vi "GEOM_findAmplifierbyCoordMult.vi"(7 "mode":enum16{"=", "<", ">", "<=", ">="}(ring), 9 "amplifiers":T1[](array[typedef]) {"fliped" items=["none", "horizontal", "vertical"]; "type" items=["LL", "LR", "UL", "UR"]}, 10 "ycoord":i32, 11 "xcoord":i32) -> (1 "amplifiers":T1[](array[typedef]) {"fliped" items=["none", "horizontal", "vertical"]; "type" items=["LL", "LR", "UL", "UR"]}, 2 "indexes":i32[](array[numeric]))   [LabVIEW 2016]
uses:
  GEOM_Amplifier.ctl
  GEOM_AmpType.ctl
  GEOM_ROI.ctl
  GEOM_Coords.ctl
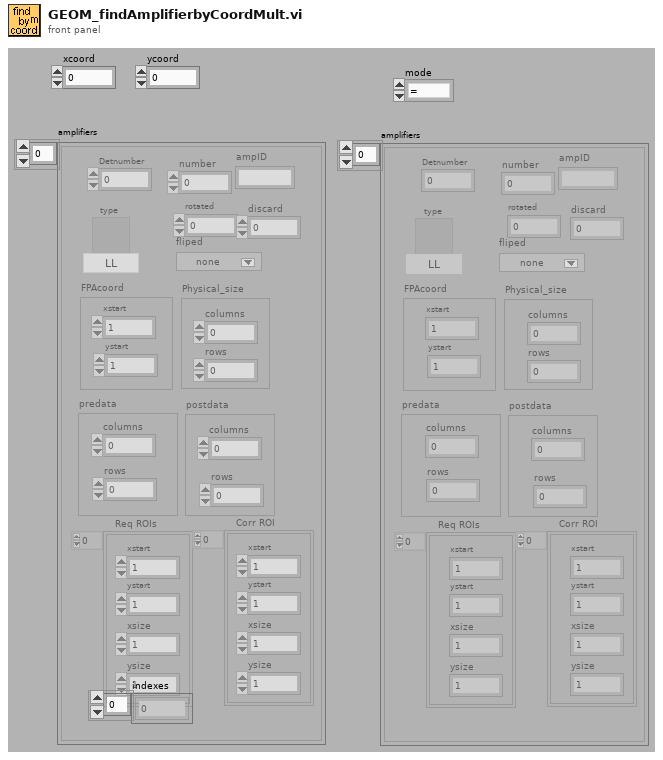
[diagram p1: front panel]
types:
  T1 = typedef "GEOM_Amplifier.ctl" = cluster{"number":i32, "type":T2, "rotated":i16, "fliped":u16, "FPAcoord":cluster{"xstart":i32, "ystart":i32}, "Physical_size":cluster{"columns":i32, "rows":i32}, "predata":cluster{"columns":i32, "rows":i32}, "postdata":cluster{"columns":i32, "rows":i32}, "Req ROIs":T3, "Corr ROI":T3, "Detnumber":i32, "ampID":string, "discard":i32}
  T2 = typedef "GEOM_AmpType.ctl" = u16
  T3 = typedef "GEOM_ROI.ctl" = T4[]
  T4 = typedef "GEOM_Coords.ctl" = cluster{"xstart":u32, "ystart":u32, "xsize":u32, "ysize":u32}
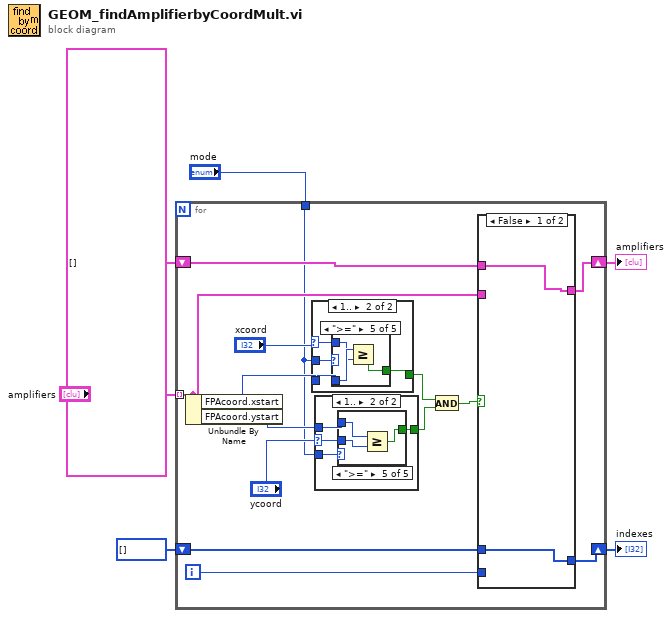
[diagram p0: block diagram]
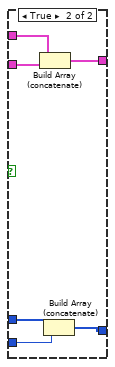
[diagram p2: hidden frame]
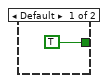
[diagram p3: hidden frame]
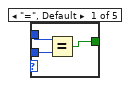
[diagram p4: hidden frame]
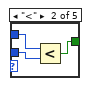
[diagram p5: hidden frame]
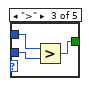
[diagram p6: hidden frame]
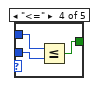
[diagram p7: hidden frame]
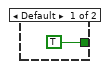
[diagram p8: hidden frame]
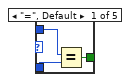
[diagram p9: hidden frame]
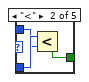
[diagram p10: hidden frame]
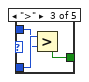
[diagram p11: hidden frame]
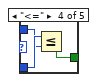
[diagram p12: hidden frame]
diagram:
  n1 = for {
    tunnel: "amplifiers" -> [w13] mode=indexing
    shift-right: [w12] -> w5
    shift-left: T1[] [] -> [w11]
    shift-right: [w9] -> w4
    shift-left: i32[] [] -> [w8]
    tunnel: "mode" -> [w7]
    i -> [w10]
    n2 = Unbundle By Name(w13) -> ("FPAcoord.xstart"=w20:i32, "FPAcoord.ystart"=w19:i32)
    n3 = case shown="1.." "xcoord" {
      selector: "xcoord" -> [_ w51]
      tunnel: w20 -> [_ w53]
      tunnel: [TRUE w52] -> w18
      tunnel: w7 -> [_ w50]
      frame Default {
      }
      frame 1.. {
        n4 = case shown="\">=\"" w50 {
          tunnel: w53 -> [w56 w58 w61 w64 w67]
          tunnel: [w55 w59 w62 w65 w68] -> w52
          tunnel: w51 -> [w54 w57 w60 w63 w66]
          frame "=", Default {
            n5 = Equal?(x=w54, y=w56) -> (x = y?=w55:bool)
          }
          frame "<" {
            n6 = Less?(x=w58, y=w57) -> (x < y?=w59:bool)
          }
          frame ">" {
            n7 = Greater?(x=w61, y=w60) -> (0:w62:bool)
          }
          frame "<=" {
            n8 = Less Or Equal?(x=w64, y=w63) -> (x <= y?=w65:bool)
          }
          frame ">=" {
            n9 = Greater Or Equal?(x=w67, y=w66) -> (x >= y?=w68:bool)
          }
        }
      }
    }
    n10 = case shown="1.." "ycoord" {
      selector: "ycoord" -> [_ w31]
      tunnel: w19 -> [_ w33]
      tunnel: [TRUE w32] -> w17
      tunnel: w7 -> [_ w30]
      frame Default {
      }
      frame 1.. {
        n11 = case shown="\">=\"" w30 {
          tunnel: w33 -> [w36 w38 w41 w44 w47]
          tunnel: [w35 w39 w42 w45 w48] -> w32
          tunnel: w31 -> [w34 w37 w40 w43 w46]
          frame "=", Default {
            n12 = Equal?(x=w36, y=w34) -> (x = y?=w35:bool)
          }
          frame "<" {
            n13 = Less?(x=w38, y=w37) -> (x < y?=w39:bool)
          }
          frame ">" {
            n14 = Greater?(x=w41, y=w40) -> (0:w42:bool)
          }
          frame "<=" {
            n15 = Less Or Equal?(x=w44, y=w43) -> (x <= y?=w45:bool)
          }
          frame ">=" {
            n16 = Greater Or Equal?(x=w47, y=w46) -> (x >= y?=w48:bool)
          }
        }
      }
    }
    n17 = And(x=w18, y=w17) -> (x .and. y?=w14:bool)
    n18 = case shown="False" w14 {
      tunnel: w13 -> [_ w28]
      tunnel: [w22 w27] -> w12
      tunnel: w11 -> [w22 w26]
      tunnel: w10 -> [_ w24]
      tunnel: [w21 w23] -> w9
      tunnel: w8 -> [w21 w25]
      frame False {
      }
      frame True {
        n19 = Build Array (concatenate)(w26, w28) -> (w27:T1[])
        n20 = Build Array (concatenate)(w25, w24) -> (w23:i32[])
      }
    }
  }
  "amplifiers" <- w5
  "indexes" <- w4
